vi "2Temperatura Random.vi"() -> ()   [LabVIEW 2016]
panel:
  in  "stop":bool
  out "Temperatura":dbl(graph)
  in  "Retardo":dbl(knob) min=0.0 max=10.0 step=1.0 scale=0.0..10.0
  in  "Numero de muestras":i32
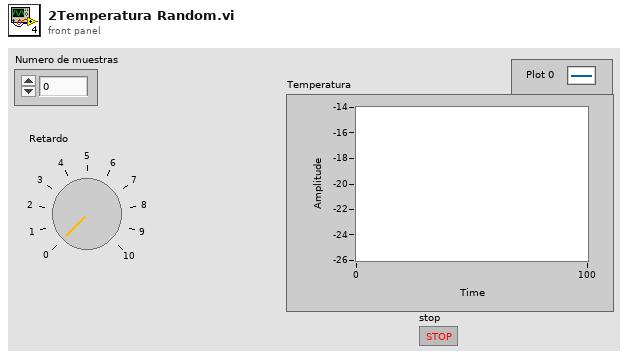
[diagram p1: front panel]
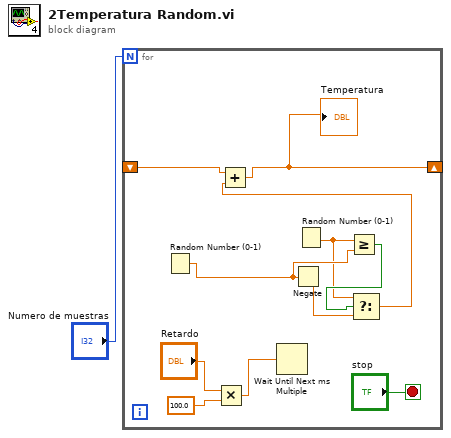
[diagram p0: block diagram]
diagram:
  n1 = for {
    N: "Numero de muestras" -> [_]
    shift-right: [w2] -> _
    shift-left: _ -> [w4]
    stop <- "stop" stop-if-true
    n2 = Random Number (0-1)() -> (number: 0 to 1=w8:dbl)
    n3 = Multiply(x="Retardo", y=100.0) -> (x*y=w10:dbl)
    n4 = Wait Until Next ms Multiple(millisecond multiple=w10) -> ()  [unwired: 1 out]
    n5 = Negate(x=w8) -> (-x=w5:dbl)
    n6 = Random Number (0-1)() -> (number: 0 to 1=w6:dbl)
    n7 = Greater Or Equal?(x=w6, y=w8) -> (x >= y?=w7:bool)
    n8 = Select(t=w6, s=w7, f=w5) -> (s? t:f=w3:dbl)
    n9 = Add(x=w4, y=w3) -> (x+y=w2:dbl)
    "Temperatura" <- w2
  }
